vi "Correct signal gen level using PM.vi"(7 "PM for power leveling":u8, 8 "error in (no error)":errorcluster, 9 "Power":dbl, 10 "Frequency":dbl, 11 "Harmonics in":refnum<class "Harmonics.lvclass">) -> (0 "error out":errorcluster, 2 "Power at DUT":dbl, 3 "Harmonics out":refnum<class "Harmonics.lvclass">)   [LabVIEW 2020, in "Harmonics.lvclass"]
uses:
  Harmonics.lvclass
  C:/Sandbox/Git_Sandbox/WiSpry Test Framework source code (LV20)/WiSpry Test Framework/Measurements/Measurement.lvclass
  Path Control/Paths.ctl
  Harmonics.lvclass/Harmonics.ctl
  Measurement.lvclass/Measurement.ctl
  Instruments/Signal Generator/Signal Generator.lvclass
  Instruments/Power Meter/Power Meter.lvclass
  Path Control/PathControl.lvclass
  Measurement.lvclass
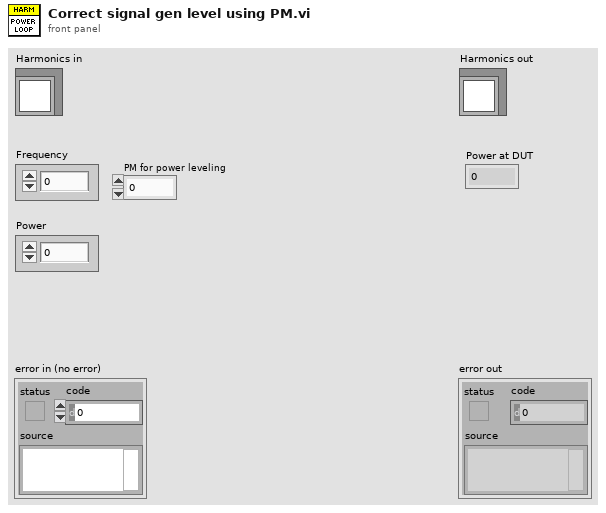
[diagram p1: front panel]
types:
  T1 = typedef "PathControl.lvclass/Paths.ctl" = enum16{"SigGen 1 -> DUT", "SigGen 2 -> DUT", "SigGen 1 -> PM 1", "SigGen 1 -> PM 2", "DUT -> SA", "DUT -> PM 2", "VSG -> DUT", "SigGen 2 -> PM 1", "SigGen 2 -> PM 2"}
  T2 = typedef "Harmonics.lvclass/Config info.ctl" = cluster{"RBW":dbl, "VBW ":dbl, "Number of Averages":i32, "Average On":bool, "Symbols":i32[], "All Harm":bool, "Loop order":T3, "Power Window":dbl, "Frequency (MHz)":string, "Power (dBm)":string, "PM for power leveling":u8, "Zero span":bool, "Stop level":dbl}
  T3 = typedef "Harmonics.lvclass/Loop order.ctl" = enum16{"Device -> Power -> Frequency", "Device -> Frequency -> Power"}
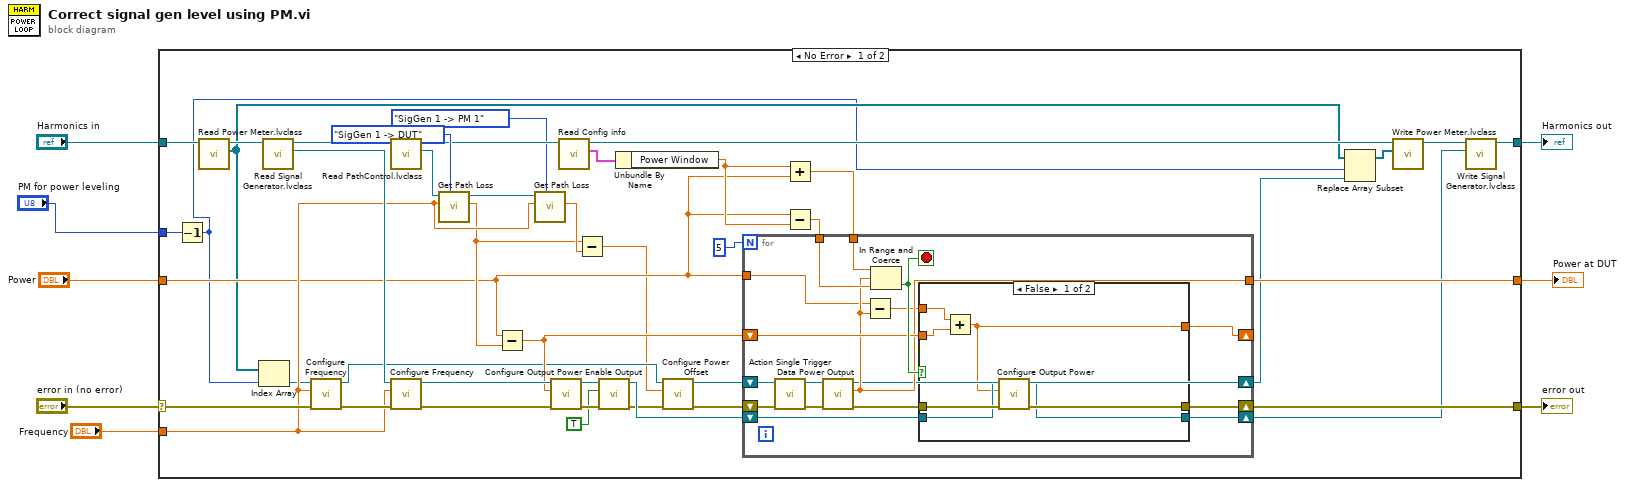
[diagram p0: block diagram]
diagram:
  n1 = case shown="No Error" "error in (no error)" {
    selector: "error in (no error)" -> [w50 w81]
    tunnel: [w28 w81] -> w7
    tunnel: [w15 w80] -> w5
    tunnel: "Harmonics in" -> [w52 w80]
    tunnel: "Frequency" -> [w43 _]
    tunnel: "Power" -> [w26 _]
    tunnel: [w20 _] -> w2
    tunnel: "PM for power leveling" -> [w10 _]
    frame No Error {
      n2 = Decrement(x=w10) -> (x-1=w9:u8)
      n3 = call "Read Power Meter.lvclass.vi"("Harmonics in"=w52) -> ("Power Meter classes"=w13:refnum<class "Power Meter.lvclass">[], "Harmonics out"=w51:refnum<class "Harmonics.lvclass">)  [unwired: 9 in]
      n4 = Index Array(array=w13, index=w9) -> (element=w18:refnum<class "Power Meter.lvclass">)
      n5 = call "Read Signal Generator.lvclass.vi"("Harmonics in"=w51) -> ("Signal Generator.lvclass"=w49:refnum<class "Signal Generator.lvclass">, "Harmonics out"=w47:refnum<class "Harmonics.lvclass">)  [unwired: 9 in]
      n6 = call-dynamic "Configure Frequency.vi"("error in (no error)"=w50, "Frequency"=w43, "Power Meter in"=w18) -> ("error out"=w48:errorcluster, "Power Meter out"=w24:refnum<class "Power Meter.lvclass">)  [unwired: 7 in]
      n7 = call "Read PathControl.lvclass.vi"("Measurements in"=w47) -> ("PathControl.lvclass"=w46:refnum<class "PathControl.lvclass">, "Measurements out"=w35:refnum<class "Harmonics.lvclass">)  [unwired: 9 in]
      n8 = call-dynamic "Configure Frequency.vi"("error in (no error)"=w48, "Frequency [Hz]"=w43, "Signal Generator in"=w49) -> ("error out"=w41:errorcluster, "Signal Generator out"=w40:refnum<class "Signal Generator.lvclass">)  [unwired: 7 in]
      n9 = call "Get Path Loss.vi"("Path"=Paths."SigGen 1 -> DUT", "Frequency [Hz]"=w43, "PathControl in"=w46) -> ("Insertion Loss (dB)"=w27:dbl, "PathControl out"=w44:refnum<class "PathControl.lvclass">)  [unwired: 5 in, 2 out]
      n10 = Subtract(x=w26, y=w27) -> (x-y=w29:dbl)
      n11 = call "Get Path Loss.vi"("Path"=Paths."SigGen 1 -> PM 1", "Frequency [Hz]"=w43, "PathControl in"=w44) -> ("Insertion Loss (dB)"=w42:dbl)  [unwired: 5 in, 3 out]
      n12 = call-dynamic "Configure Output Power.vi"("error in (no error)"=w41, "Output Power [dBm]"=w29, "Signal Generator in"=w40) -> ("error out"=w39:errorcluster, "Signal Generator out"=w38:refnum<class "Signal Generator.lvclass">)  [unwired: 7 in]
      n13 = call "Read Config info.vi"("Harmonics in"=w35) -> ("Config info"=w34:T2, "Harmonics out"=w16:refnum<class "Harmonics.lvclass">)  [unwired: 9 in]
      n14 = Subtract(x=w27, y=w42) -> (x-y=w22:dbl)
      n15 = call-dynamic "Enable Output.vi"("error in (no error)"=w39, "Output Enable (F)"=TRUE, "Signal Generator in"=w38) -> ("error out"=w21:errorcluster, "Signal Generator out"=w36:refnum<class "Signal Generator.lvclass">)  [unwired: 7 in]
      n16 = Unbundle By Name(w34) -> ("Power Window"=w33:dbl)
      n17 = call-dynamic "Configure Power Offset.vi"("error in (no error)"=w21, "Power Offset"=w22, "Power Meter in"=w24) -> ("error out"=w25:errorcluster, "Power Meter out"=w23:refnum<class "Power Meter.lvclass">)  [unwired: 7 in]
      n18 = Add(x=w33, y=w26) -> (x+y=w32:dbl)
      n19 = Subtract(x=w26, y=w33) -> (x-y=w31:dbl)
      n20 = for {
        N: 5 -> [_]
        shift-right: [w61] -> w28
        shift-left: w25 -> [w69]
        tunnel: w32 -> [w64]
        tunnel: w31 -> [w65]
        tunnel: [w59] -> w20
        shift-right: [w56] -> _
        shift-left: w29 -> [w60]
        tunnel: w26 -> [w55]
        shift-right: [w54] -> w14
        shift-left: w36 -> [w57]
        shift-right: [w53] -> w11
        shift-left: w23 -> [w68]
        stop <- w63 stop-if-true
        n21 = call-dynamic "Action Single Trigger.vi"("error in (no error)"=w69, "Power Meter in"=w68) -> ("error out"=w67:errorcluster, "Power Meter out"=w66:refnum<class "Power Meter.lvclass">)  [unwired: 8 in]
        n22 = call-dynamic "Data Power Output.vi"("error in (no error)"=w67, "Power Meter in"=w66) -> ("error out"=w62:errorcluster, "Power Out"=w59:dbl, "Power Meter out"=w53:refnum<class "Power Meter.lvclass">)  [unwired: 7 in]
        n23 = Subtract(x=w55, y=w59) -> (x-y=w58:dbl)
        n24 = In Range and Coerce(upper limit=w64, x=w59, lower limit=w65) -> (In Range?=w63:bool)  [unwired: 1 out]
        n25 = case shown="False" w63 {
          tunnel: w62 -> [w74 w79]
          tunnel: [w71 w79] -> w61
          tunnel: w60 -> [w76 w78]
          tunnel: w58 -> [w75 _]
          tunnel: w57 -> [w73 w77]
          tunnel: [w72 w78] -> w56
          tunnel: [w70 w77] -> w54
          frame False {
            n26 = Add(x=w75, y=w76) -> (x+y=w72:dbl)
            n27 = call-dynamic "Configure Output Power.vi"("error in (no error)"=w74, "Output Power [dBm]"=w72, "Signal Generator in"=w73) -> ("error out"=w71:errorcluster, "Signal Generator out"=w70:refnum<class "Signal Generator.lvclass">)  [unwired: 7 in]
          }
          frame True {
          }
        }
      }
      n28 = Replace Array Subset(array=w13, new element=w11, index=w9) -> (w12:refnum<class "Power Meter.lvclass">[])
      n29 = call "Write Power Meter.lvclass.vi"("Power Meter classes"=w12, "Harmonics in"=w16) -> ("Harmonics out"=w17:refnum<class "Harmonics.lvclass">)  [unwired: 9 in]
      n30 = call "Write Signal Generator.lvclass.vi"("Signal Generator.lvclass"=w14, "Harmonics in"=w17) -> ("Harmonics out"=w15:refnum<class "Harmonics.lvclass">)  [unwired: 9 in]
    }
    frame Error {
    }
  }
  "error out" <- w7
  "Harmonics out" <- w5
  "Power at DUT" <- w2
